vi "_ClassFieldsEditor_Interface.vi"(9 "EventsIn":T1, 10 "Events":T2) -> ()   [LabVIEW 2014, in "_ClassFieldsEditor.lvclass"]
uses:
  _ClassFieldsEditor.lvclass
  GCMCore/Providers/Veritech_GCM/Support/Framework/_Plugins/_LVCMPlugin/GCMPlugin_EventsOut.ctl
  GCMCore/Providers/Veritech_GCM/Support/Framework/_Plugins/_LVCMPlugin/GCMPlugin_EventsIn.ctl
  ClassFieldsEditor_States.ctl
  ClassFieldsEditor_Data.ctl
  <vilib>/Utility/VariantDataType/VariantType.lvlib
  <resource>/Framework/Providers/LVClassLibrary/NewAccessors/MemberVICreation.lvlib
  GCMCore/Providers/Veritech_GCM/Support/Framework/_Plugins/GCMPlugin/GCMPlugin.lvclass
panel:
  in  "Cancel":bool
  in  "Ok 2":bool
  in  "New Accesor":bool
  in  "Fields":i32(listbox)
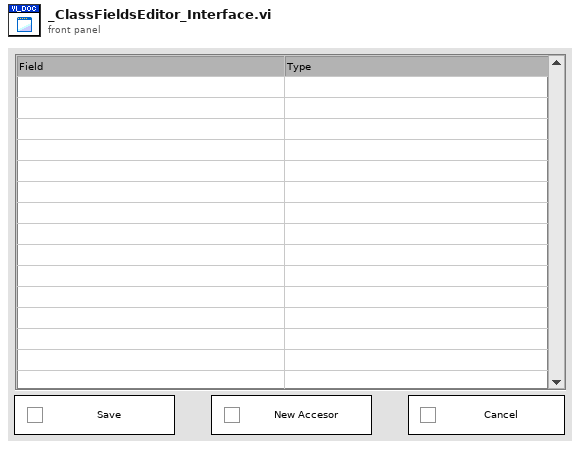
[diagram p1: front panel]
types:
  T1 = typedef "GCMPlugin.lvclass/GCMPlugin_EventsIn.ctl" = cluster{"Stop":refnum<user-event>, "ItemSelected":refnum<user-event>, "ItemDeselected":refnum<user-event>, "PluginActivated":refnum<user-event>, "PluginDeactivated":refnum<user-event>}
  T2 = typedef "GCMPlugin.lvclass/GCMPlugin_EventsOut.ctl" = cluster{"ItemEdited":refnum<user-event>}
  T3 = typedef "_ClassFieldsEditor.lvclass/ClassFieldsEditor_Data.ctl" = cluster{"Controls":refnum<vi>[]}
  T4 = typedef "_ClassFieldsEditor.lvclass/ClassFieldsEditor_States.ctl" = enum16{"Init", "WaitForEvent", "Stop"}
  T5 = typedef "VariantType.lvlib/Type.ctl" = enum8{"Invalid Type", "Void", "I8", "I16", "I32", "I64", "U8", "U16", "U32", "U64", "Single Float", "Double Float", "Extended Float", "Single Complex", "Double Complex", "Extended Complex", "Enum U8", "Enum U16", "Enum U32", "Enum U64", "Single Float With Unit", "Double Float With Unit", "Extended Float With Unit", "Single Complex with Unit", "Double Complex with Unit", "Extended Complex with Unit", "Boolean", "String", "Path", "Picture", "Tag", "Array", "Cluster", "Variant", "LV Variant", "Waveform", "Timestamp", "Digital Waveform", "Digital Data", "ExpressData", "Refnum", "External Data", "VI", "Poly VI", "LabVIEW Class Instance", "Fixed Point"}
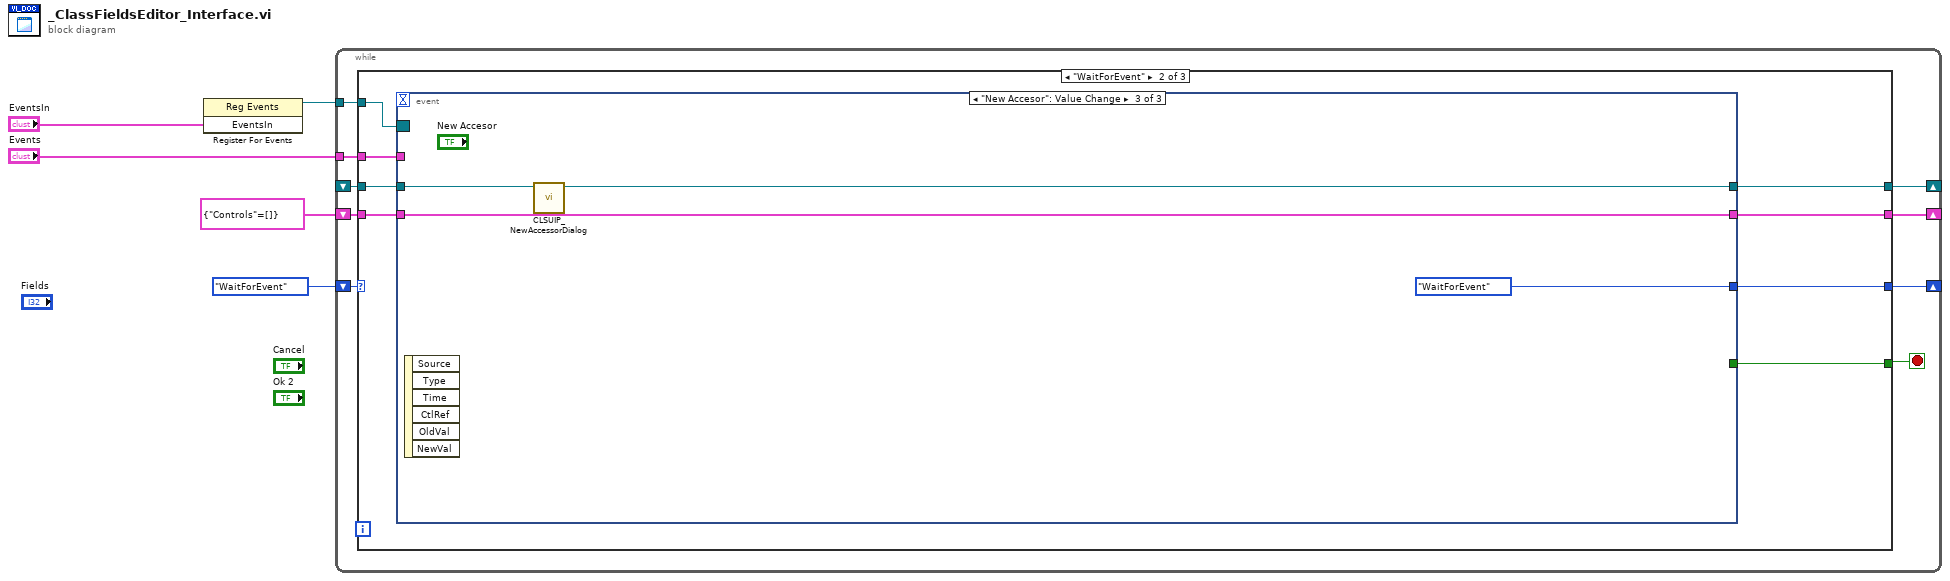
[diagram p0: block diagram]
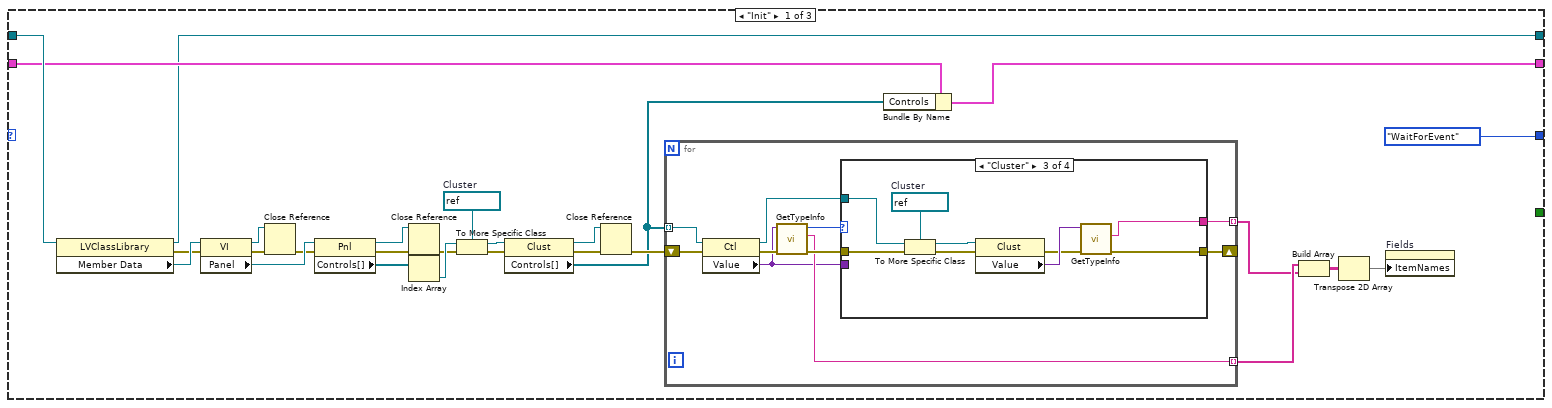
[diagram p2: hidden frame]
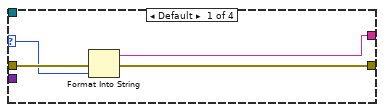
[diagram p3: hidden frame]
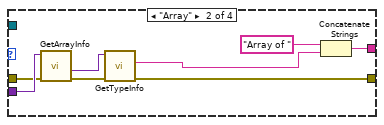
[diagram p4: hidden frame]
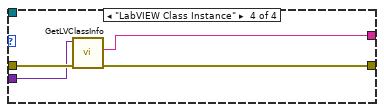
[diagram p5: hidden frame]
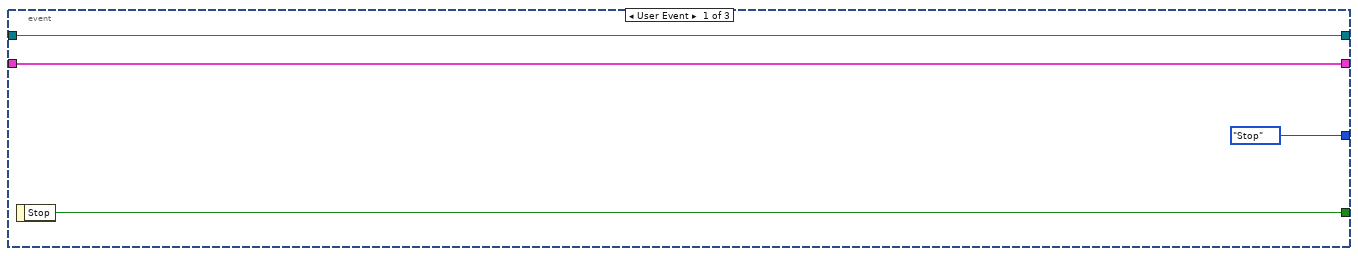
[diagram p6: hidden frame]
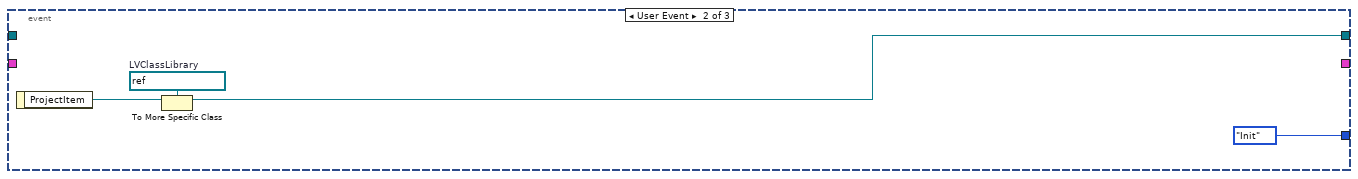
[diagram p7: hidden frame]
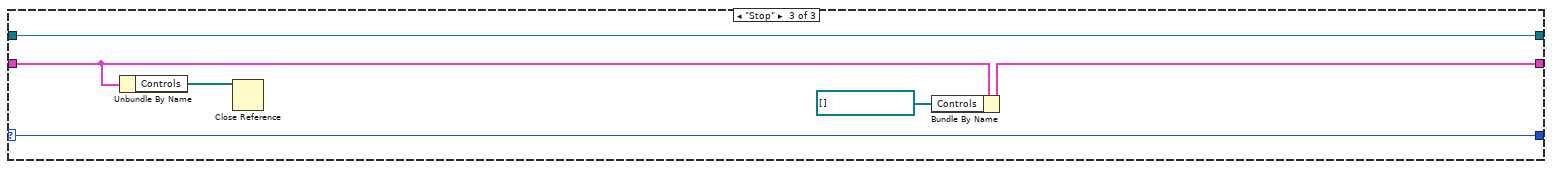
[diagram p8: hidden frame]
diagram:
  n1 = register-events("EventsIn") -> (reference out=w4:refnum<event-registration>)  [unwired: 2 in, 1 out]
  n2 = while {
    tunnel: w4 -> [w14]
    tunnel: "Events" -> [w13]
    shift-right: [w9] -> _
    shift-left: ClassFieldsEditor_States."WaitForEvent" -> [w11]
    shift-right: [w7] -> _
    shift-left: T3 {"Controls"=[]} ("FieldsEditorData") -> [w8]
    shift-right: [w6] -> _
    shift-left: _ -> [w10]
    stop <- w12 stop-if-true
    n3 = case shown="\"WaitForEvent\"" w11 {
      selector: w11 -> [_ _ w102]
      tunnel: w14 -> [_ w84 _]
      tunnel: w13 -> [_ w83 _]
      tunnel: [_ w82 _] -> w12
      tunnel: w10 -> [w38 w81 w97]
      tunnel: [ClassFieldsEditor_States."WaitForEvent" w78 w102] -> w9
      tunnel: w8 -> [w17 w79 w101]
      tunnel: [w16 w80 w100] -> w7
      tunnel: [w15 w77 w97] -> w6
      frame "Init" {
        w37 = refnum<vi> refnum  # Cluster
        n4 = property class="LVClassLibrary"(reference=w38) -> (reference out=w15:refnum<vi>, error out=w29:errorcluster, "Member Data"=w39:refnum<vi>)  [unwired: 1 in]
        n5 = property class="VI"(reference=w39, error in=w29) -> (reference out=w24:refnum<vi>, error out=w28:errorcluster, "Panel"=w40:refnum<vi>)
        n6 = Close Reference(reference=w24, error in (no error)=w28) -> (error out=w27:errorcluster)
        n7 = property class="Pnl"(reference=w40, error in=w27) -> (reference out=w22:refnum<vi>, error out=w23:errorcluster, "Controls[]"=w41:refnum<vi>[])
        n8 = Close Reference(reference=w22, error in (no error)=w23) -> (error out=w21:errorcluster)
        n9 = Index Array(array=w41) -> (element=w35:refnum<vi>)  [unwired: 1 in]
        n10 = To More Specific Class(target class=w37, reference=w35, error in=w21) -> (specific class reference=w36:refnum<vi>, error out=w26:errorcluster)
        n11 = property class="Clust"(reference=w36, error in=w26) -> (reference out=w19:refnum<vi>, error out=w25:errorcluster, "Controls[]"=w18:refnum<vi>[])
        n12 = Close Reference(reference=w19, error in (no error)=w25) -> (error out=w20:errorcluster)
        n13 = for {
          tunnel: w18 -> [w49] mode=indexing
          tunnel: [w51] -> w32 mode=indexing
          tunnel: [w43] -> w33 mode=indexing
          shift-right: [w50] -> _
          shift-left: w20 -> [w48]
          n14 = property class="Ctl"(reference=w49, error in=w48) -> (reference out=w46:refnum<vi>, error out=w47:errorcluster, "Value"=w42:variant)
          n15 = call <vilib>:"GetTypeInfo.vi"("error in (no error)"=w47, "Variant"=w42) -> ("error out"=w45:errorcluster, "Name"=w43:string, "Type Enum"=w44:T5)  [unwired: 5 in, 2 out]
          n16 = case shown="\"Cluster\"" w44 {
            selector: w44 -> [w54 _ _ _]
            tunnel: w46 -> [_ _ w71 _]
            tunnel: [w52 w62 w70 w73] -> w51
            tunnel: w45 -> [w55 w60 w64 w76]
            tunnel: [w53 w56 w67 w74] -> w50
            tunnel: w42 -> [_ w61 _ w75]
            frame Default {
              n17 = Format Into String(error in=w55, w54) -> (resulting string=w52:string, error out=w53:errorcluster)  [unwired: 2 in]
            }
            frame "Array" {
              n18 = call <vilib>:"GetArrayInfo.vi"("error in (no error)"=w60, "Variant"=w61) -> ("error out"=w58:errorcluster, "ArrayElement"=w59:variant)  [unwired: 6 in, 2 out]
              n19 = call <vilib>:"GetTypeInfo.vi"("error in (no error)"=w58, "Variant"=w59) -> ("error out"=w56:errorcluster, "Name"=w57:string)  [unwired: 5 in, 3 out]
              n20 = Concatenate Strings("Array of " ("string"), w57) -> (w62:string)
            }
            frame "Cluster" {
              w72 = refnum<vi> refnum  # Cluster
              n21 = To More Specific Class(target class=w72, reference=w71, error in=w64) -> (specific class reference=w69:refnum<vi>, error out=w65:errorcluster)
              n22 = property class="Clust"(reference=w69, error in=w65) -> (error out=w66:errorcluster, "Value"=w68:variant)  [unwired: 1 out]
              n23 = call <vilib>:"GetTypeInfo.vi"("error in (no error)"=w66, "Variant"=w68) -> ("error out"=w67:errorcluster, "Name"=w70:string)  [unwired: 5 in, 3 out]
            }
            frame "LabVIEW Class Instance" {
              n24 = call <vilib>:"GetLVClassInfo.vi"("error in (no error)"=w76, "Variant"=w75) -> ("error out"=w74:errorcluster, "LV Class File Name"=w73:string)  [unwired: 7 in, 1 out]
            }
          }
        }
        n25 = Bundle By Name(cluster=w17, "Controls"=w18) -> (w16:T3)
        n26 = Build Array(w33, w32) -> (w31:string[][])
        n27 = Transpose 2D Array(2D array=w31) -> (transposed array=w30:string[][])
        n28 = property on="Fields" class="MCListbox (strict)"("ItemNames"=w30) -> ()  [unwired: 2 in, 2 out]
      }
      frame "WaitForEvent" {
        n29 = event shown="[2] \"New Accesor\": Value Change" {
          selector: w84 -> [_ _ _]
          dyn-events: _ -> [_ _ _]
          timeout: _ -> [_ _ _]
          tunnel: w83 -> [_ _ _]
          tunnel: [w88 _ _] -> w82
          tunnel: w81 -> [w85 _ w96]
          tunnel: [w87 _ w95] -> w80
          tunnel: w79 -> [w87 _ w95]
          tunnel: [ClassFieldsEditor_States."Stop" ClassFieldsEditor_States."Init" ClassFieldsEditor_States."WaitForEvent"] -> w78
          tunnel: [w85 w90 w93] -> w77
          event User Event {
            n30 = event-data() -> ("Stop"=w88:bool)  [unwired: 1 in]
          }
          event User Event {
            w92 = refnum<vi> refnum  # LVClassLibrary
            n31 = event-data() -> ("ProjectItem"=w91:refnum<vi>)  [unwired: 1 in]
            n32 = To More Specific Class(target class=w92, reference=w91) -> (specific class reference=w90:refnum<vi>)  [unwired: 1 in, 1 out]
          }
          event "New Accesor": Value Change {
            n33 = event-data() -> ()  [unwired: 1 in, 6 out]
            n34 = call <resource>:"CLSUIP_NewAccessorDialog.vi"("DNL_LVClassLibrary Refnum"=w96) -> ("DNL_LVClassLibrary Refnum out"=w93:refnum<vi>)  [unwired: 8 in, 2 out]
          }
        }
      }
      frame "Stop" {
        n35 = Unbundle By Name(w101) -> ("Controls"=w98:refnum<vi>[])
        n36 = Close Reference(reference=w98) -> ()  [unwired: 1 in, 1 out]
        n37 = Bundle By Name(cluster=w101, "Controls"=refnum<vi>[] []) -> (w100:T3)
      }
    }
  }
